vi "GEA3 Send Data ERD.vi"(8 "error in (no error)":errorcluster, 10 "ERD Write Data In":T2 {"ERD Number" format="%.0x"}, 11 ".NET Refnum in":refnum<k24>) -> (0 "error out":errorcluster, 1 "GEA Message":T1 {"Command" format="%02x"; "Destination" format="%02x"; "Source" format="%02x"}, 2 "Raw Data Out":string, 3 "GEA2 Reference Out":refnum<k24>)   [LabVIEW 2019]
uses:
  type defs/ERD Write Data In.ctl
  type defs/Data Type.ctl
  C:/TechnologyLab/NI-2010/Drivers/GEA3 Toolkit/GEA3 DLL Source/GeaCommunication.dll
  GEA3 DLL Source/GeaCommunication.dll
  type defs/Data In.ctl
  library/GEA2_Toolkit.lvlib
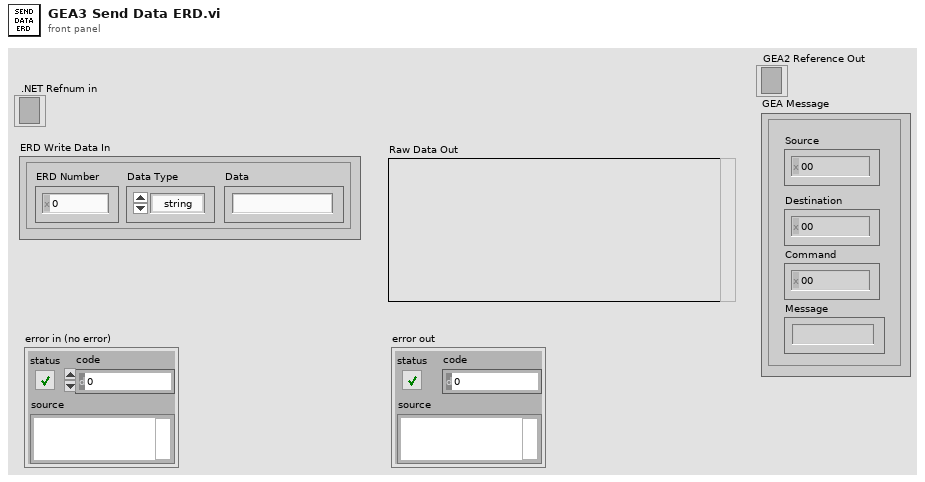
[diagram p1: front panel]
types:
  T1 = typedef "GEA2_Toolkit.lvlib/Data In.ctl" = cluster{"Source":u8, "Destination":u8, "Command":u8, "Message":string}
  T2 = typedef "GEA2_Toolkit.lvlib/ERD Write Data In.ctl" = cluster{"ERD Number":u16, "Data Type":T3, "Data":string}
  T3 = typedef "GEA2_Toolkit.lvlib/Data Type.ctl" = enum16{"string", "boolean", "uint8_t", "uint16_t", "uint32_t", "uint64_t", "int8_t", "int16_t", "int32_t", "int64_t"}
  T4 = typedef "GEA2_Toolkit.lvlib/Source_Destination.ctl" = cluster{"Source":u8, "Destination":u8}
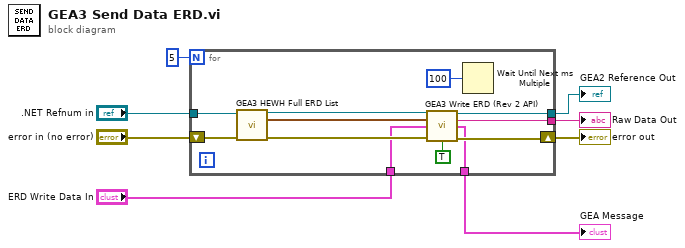
[diagram p0: block diagram]
diagram:
  n1 = for {
    N: 5 -> [_]
    tunnel: ".NET Refnum in" -> [w13]
    shift-right: [w14] -> w5
    shift-left: "error in (no error)" -> [w15]
    tunnel: "ERD Write Data In" -> [w12]
    tunnel: [w11] -> w3
    tunnel: [w10] -> w2
    tunnel: [w9] -> w1
    n2 = call "GEA3 HEWH Full ERD List.vi"("GEA2 Reference In"=w13, "error in (no error)"=w15) -> ("GEA2 Reference Out"=w16:refnum<k24>, "GEA Inputs"=w17:T4, "error out"=w18:errorcluster)  [unwired: 9 in, 2 out]
    n3 = call "GEA3 Write ERD (Rev 2 API).vi"("GEA2 Reference In"=w16, "GEA Inputs"=w17, "ERD Write Data In"=w12, "Error In"=w18, "Verify ERD Response?"=TRUE) -> ("GEA2 Reference Out"=w10:refnum<k24>, "Raw Data Out"=w11:string, "GEA Message"=w9:T1, "Error Out"=w14:errorcluster)  [unwired: 7 in]
    n4 = Wait Until Next ms Multiple(millisecond multiple=u32 100) -> ()  [unwired: 1 out]
  }
  "error out" <- w5
  "Raw Data Out" <- w3
  "GEA2 Reference Out" <- w2
  "GEA Message" <- w1
